vi "Save_Max_and_Min_Values.vi"() -> (5 "Plug in titles":string[](array[string]), 7 "Plug in values":string[](array[string]))   [LabVIEW 2010]
uses:
  Globals/Meas_global.vi
  Globals/Plug_in_data_global.vi
panel:
  in  "No of Points to average over":i32=2 min=1 step=1
  out "Minimums":dbl[](array[numeric]) format="%.2f"
  out "Maximums":dbl[](array[numeric]) format="%.2f"
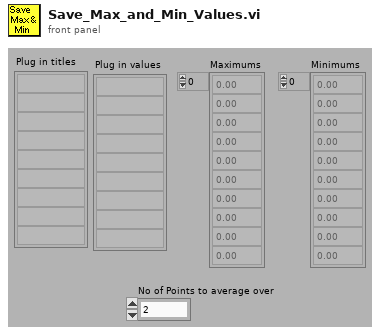
[diagram p1: front panel]
types:
  T1 = typedef "Analysis_info_cluster.ctl" = cluster{"Colour":u32, "Inst type":T2, "Inst name":string, "Symbol":string, "Code name":string, "Extra Info":string, "Inst Array":T3, "Index":i32, "Voltage Index":i32, "Extra Titles":string[], "Extra Values":string[]}
  T2 = typedef "Inst_type.ctl" = enum16{"Propeller anemometer", "Raw voltage", "Pressure Transducer", "Pitot-static tube", "Preston tube", "Hot wire", "Cross wire 1", "Cross wire 2", "Generic Linear", "Generic Polynomial", "Generic BackPoly", "Fast FID", "Thermocouple", "Cold wire", "Pulsed Wire", "LDA Vel", "LDA Tran time", "LDA Arr time"}
  T3 = typedef "Instrument_Array.ctl" = enum16{"PWA", "LDA", "Analogue"}
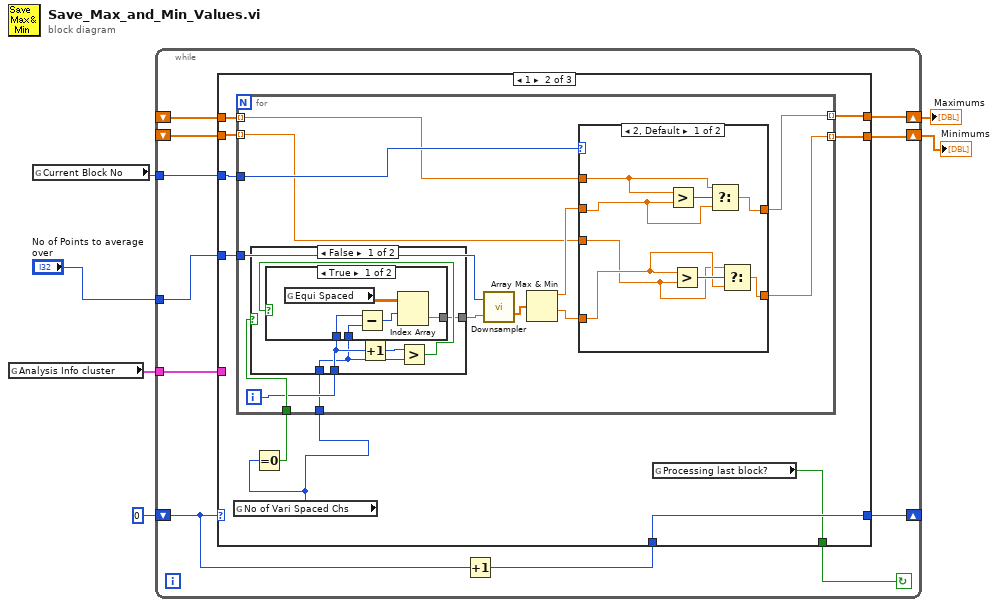
[diagram p0: block diagram]
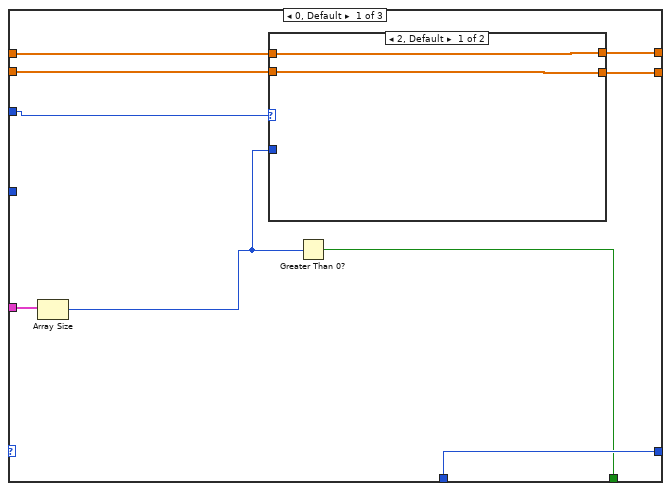
[diagram p2: hidden frame]
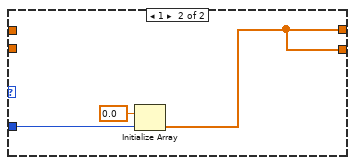
[diagram p3: hidden frame]
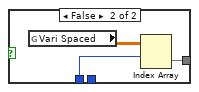
[diagram p4: hidden frame]
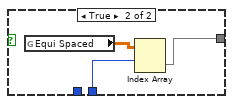
[diagram p5: hidden frame]
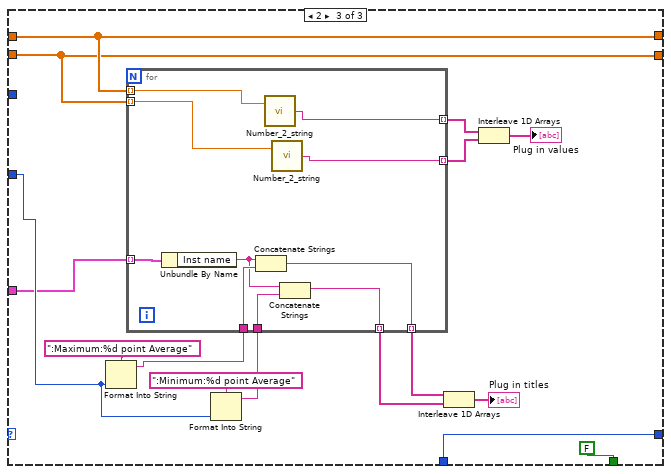
[diagram p7: hidden frame]
diagram:
  n1 = global read "Meas_global.vi" "Analysis Info cluster"() -> (w1:T1[])
  n2 = global read "Meas_global.vi" "Current Block No"() -> (w6:i32)
  n3 = while {
    shift-left: _ -> [w11]
    shift-right: [w12] -> w4
    shift-left: _ -> [w9]
    shift-right: [w10] -> w3
    shift-left: 0 -> [w16]
    shift-right: [w14] -> _
    tunnel: w6 -> [w17]
    tunnel: "No of Points to average over" -> [w8]
    tunnel: w1 -> [w7]
    stop <- w13 continue-if-true
    n4 = Increment(x=w16) -> (x+1=w15:i32)
    n5 = case shown="1" w16 {
      tunnel: w17 -> [w24 w41 _]
      tunnel: w15 -> [w26 w40 w95]
      tunnel: [w26 w40 w95] -> w14
      tunnel: [w25 w35 FALSE] -> w13
      tunnel: [w23 w37 w88] -> w12
      tunnel: w11 -> [w22 w39 w88]
      tunnel: [w21 w36 w87] -> w10
      tunnel: w9 -> [w20 w38 w87]
      tunnel: w8 -> [_ w34 w84]
      tunnel: w7 -> [w19 _ w81]
      frame 0, Default {
        n6 = Array Size(array=w19) -> (size(s)=w18:i32)
        n7 = case shown="2, Default" w24 {
          tunnel: [w28 w29] -> w23
          tunnel: w22 -> [w28 _]
          tunnel: [w27 w29] -> w21
          tunnel: w20 -> [w27 _]
          tunnel: w18 -> [_ w31]
          frame 2, Default {
          }
          frame 1 {
            n8 = Initialize Array(0.0 ("Element Data"), w31) -> (w29:dbl[])
          }
        }
        n9 = Greater Than 0?(x=w18) -> (x > 0?=w25:bool)
      }
      frame 1 {
        n10 = global read "Meas_global.vi" "No of Vari Spaced Chs"() -> (w32:i32)
        n11 = Equal To 0?(x=w32) -> (x = 0?=w33:bool)
        n12 = for {
          tunnel: w41 -> [w52]
          tunnel: w39 -> [w51] mode=indexing
          tunnel: w38 -> [w50] mode=indexing
          tunnel: [w49] -> w37 mode=indexing
          tunnel: [w48] -> w36 mode=indexing
          tunnel: w34 -> [w46]
          tunnel: w33 -> [w45]
          tunnel: w32 -> [w42]
          i -> [w44]
          n13 = case shown="False" w45 {
            tunnel: w44 -> [w58 w69]
            tunnel: [w56 w68] -> w43
            tunnel: w42 -> [w57 _]
            frame False {
              n14 = Increment(x=w58) -> (x+1=w55:i32)
              n15 = Greater?(x=w55, y=w57) -> (0:w59:bool)
              n16 = case shown="True" w59 {
                tunnel: w58 -> [w63 w65]
                tunnel: w57 -> [w62 _]
                tunnel: [w60 w66] -> w56
                frame True {
                  n17 = global read "Plug_in_data_global.vi" "Equi Spaced"() -> (w64:dbl[][])
                  n18 = Subtract(x=w63, y=w62) -> (x-y=w61:i32)
                  n19 = Index Array(array=w64, index (row)=w61) -> (element=w60:dbl[])  [unwired: 1 in]
                }
                frame False {
                  n20 = global read "Plug_in_data_global.vi" "Vari Spaced"() -> (w67:dbl[][])
                  n21 = Index Array(array=w67, index (row)=w65) -> (element=w66:dbl[])  [unwired: 1 in]
                }
              }
            }
            frame True {
              n22 = global read "Plug_in_data_global.vi" "Equi Spaced"() -> (w70:dbl[][])
              n23 = Index Array(array=w70, index (row)=w69) -> (element=w68:dbl[])  [unwired: 1 in]
            }
          }
          n24 = call "Downsampler.vi"("Input Array"=w43, "Averaging samples"=w46) -> ("Downsampled Array"=w47:dbl[])  [unwired: 1 out]
          n25 = Array Max & Min(array=w47) -> (max value=w54:dbl, min value=w53:dbl)  [unwired: 2 out]
          n26 = case shown="2, Default" w52 {
            tunnel: [w76 w80] -> w49
            tunnel: w54 -> [w77 w80]
            tunnel: [w73 w79] -> w48
            tunnel: w53 -> [w74 w79]
            tunnel: w51 -> [w72 _]
            tunnel: w50 -> [w71 _]
            frame 2, Default {
              n27 = Greater?(x=w72, y=w77) -> (0:w78:bool)
              n28 = Greater?(x=w74, y=w71) -> (0:w75:bool)
              n29 = Select(t=w72, s=w78, f=w77) -> (s? t:f=w76:dbl)
              n30 = Select(t=w71, s=w75, f=w74) -> (s? t:f=w73:dbl)
            }
            frame 1 {
            }
          }
        }
        n31 = global read "Meas_global.vi" "Processing last block?"() -> (w35:bool)
      }
      frame 2 {
        n32 = Format Into String(format string=":Maximum:%d point Average", w84) -> (resulting string=w82:string)  [unwired: 2 in, 1 out]
        n33 = Format Into String(format string=":Minimum:%d point Average", w84) -> (resulting string=w83:string)  [unwired: 2 in, 1 out]
        n34 = for {
          tunnel: w81 -> [w106] mode=indexing
          tunnel: w82 -> [w105]
          tunnel: w83 -> [w103]
          tunnel: [w102] -> w94 mode=indexing
          tunnel: [w101] -> w93 mode=indexing
          tunnel: w88 -> [w100] mode=indexing
          tunnel: w87 -> [w99] mode=indexing
          tunnel: [w97] -> w91 mode=indexing
          tunnel: [w98] -> w90 mode=indexing
          n35 = Unbundle By Name(w106) -> ("Inst name"=w104:string)
          n36 = Concatenate Strings(w104, w105) -> (w102:string)
          n37 = call "Number_2_string.vi"("number"=w100) -> ("String"=w97:string)  [unwired: 1 in]
          n38 = call "Number_2_string.vi"("number"=w99) -> ("String"=w98:string)  [unwired: 1 in]
          n39 = Concatenate Strings(w104, w103) -> (w101:string)
        }
        n40 = Interleave 1D Arrays(w94, w93) -> (→"Plug in titles":string[])
        n41 = Interleave 1D Arrays(w91, w90) -> (→"Plug in values":string[])
      }
    }
  }
  "Maximums" <- w4
  "Minimums" <- w3
